vi "Finalize To Settings.vi"(8 "error in (no error)":errorcluster, 11 "Core Transfer Configuration in":refnum<class "Transfer Configuration.lvclass">) -> (0 "error out":errorcluster, 2 "settings":cluster{"key":string, "value":string}[](array[cluster]), 3 "Core Transfer Configuration out":refnum<class "Transfer Configuration.lvclass">)   [LabVIEW 2019, in "DSF Core.lvlib" / "Transfer Configuration.lvclass"]
uses:
  Transfer Configuration.lvclass
  Transfer Configuration.lvclass/Transfer Configuration.ctl
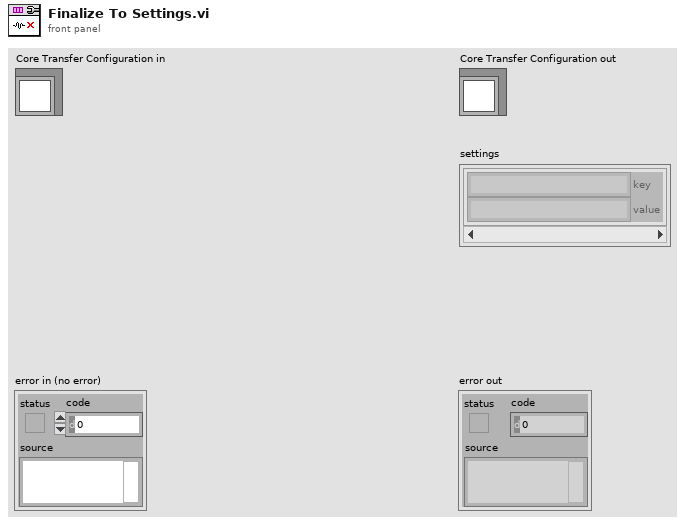
[diagram p1: front panel]
types:
  T1 = typedef "DSF Core.lvlib/Transfer Configuration.lvclass/Core Transfer Configuration.ctl" = cluster{"name":string}
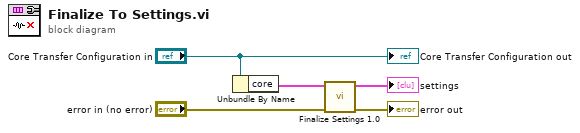
[diagram p0: block diagram]
diagram:
  n1 = Unbundle By Name("Core Transfer Configuration in") -> ("core"=w2:T1)
  n2 = call "Finalize Settings 1.0.vi"("error in (no error)"="error in (no error)", "configuration 1.0"=w2) -> ("error out"=→"error out":errorcluster, "settings 1.0"=→"settings":cluster{"key":string, "value":string}[])  [unwired: 7 in, 1 out]
  "Core Transfer Configuration out" <- "Core Transfer Configuration in"
